vi "RX Disabled channel logic 2ch 4SPC.vi"(7 "reset":bool, 9 "input valid":bool, 10 "U32 data in":u32[](array[numeric])=[0, 0, 0, 0, 0, 0, 0, 0], 11 "enabled channels":u32) -> (1 "data ready":bool, 2 "U32 data out":u32[](array[numeric]))   [LabVIEW 2025, in "niUSRP Stream Control (DMA) v1 FPGA.lvclass"]
uses:
  niUSRP Stream Control (DMA) v1 FPGA.lvclass
  niUSRP Stream Control (DMA) v1 FPGA.lvclass/niUSRP Stream Control (DMA) v1 FPGA.ctl
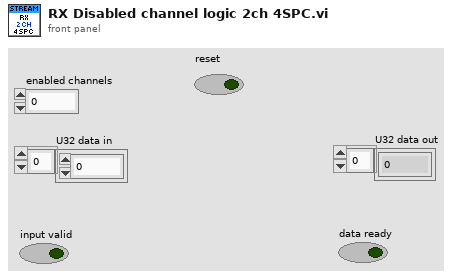
[diagram p1: front panel]
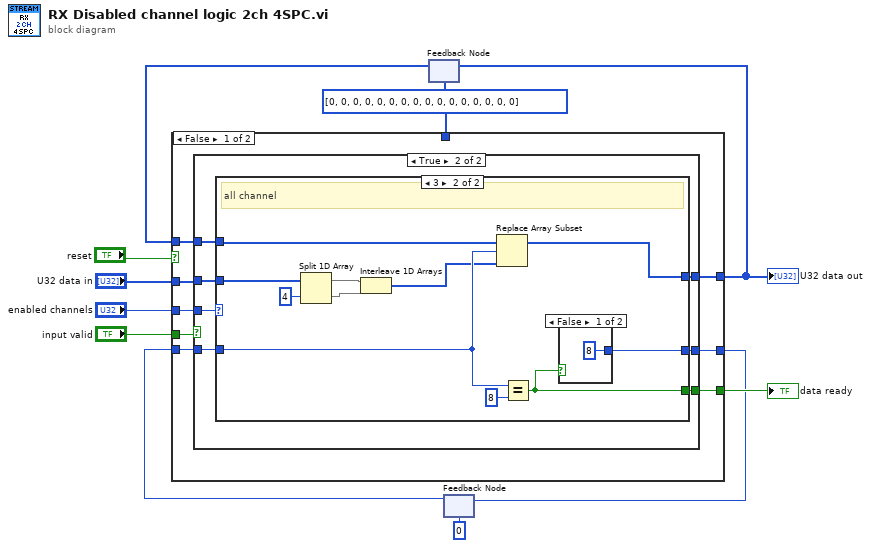
[diagram p0: block diagram]
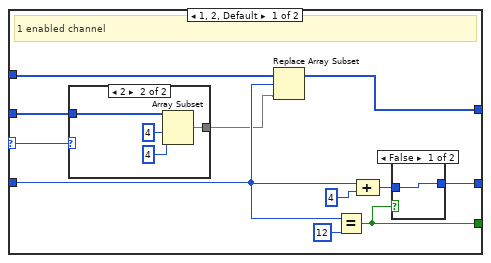
[diagram p3: hidden frame]
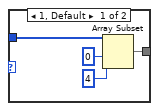
[diagram p4: hidden frame]
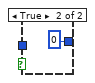
[diagram p5: hidden frame]
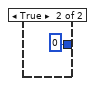
[diagram p6: hidden frame]
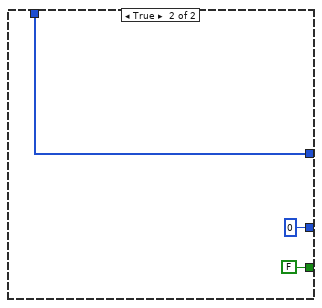
[diagram p7: hidden frame]
diagram:
  w1 = u32[] [0, 0, 0, 0, 0, 0, 0, 0, 0, 0, 0, 0, 0, 0, 0, 0]
  n1 = feedback #1(w1) -> (w11:u32[])
  n2 = feedback #2(u8 0) -> (w5:u8)
  n3 = case shown="False" "reset" {
    tunnel: w11 -> [w19 _]
    tunnel: "input valid" -> [w18 _]
    tunnel: "U32 data in" -> [w17 _]
    tunnel: [w16 w64] -> w8
    tunnel: "enabled channels" -> [w15 _]
    tunnel: w5 -> [w14 _]
    tunnel: [w13 FALSE] -> w4
    tunnel: [w12 u8 0] -> w3
    tunnel: w1 -> [_ w64]
    frame False {
      n4 = case shown="True" w18 {
        selector: w18 -> [w22 _]
        tunnel: w19 -> [w20 w29]
        tunnel: w15 -> [_ w28]
        tunnel: w17 -> [_ w27]
        tunnel: w14 -> [w21 w26]
        tunnel: [w20 w25] -> w16
        tunnel: [w21 w24] -> w12
        tunnel: [w22 w23] -> w13
        frame False {
        }
        frame True {
          n5 = case shown="3" w28 {
            selector: w28 -> [w31 _]
            tunnel: w27 -> [w32 w52]
            tunnel: [w39 w56] -> w25
            tunnel: [w35 w58] -> w23
            tunnel: w26 -> [w37 w59]
            tunnel: [w34 w57] -> w24
            tunnel: w29 -> [w38 w60]
            frame 1, 2, Default {
              # "1 enabled channel"
              n6 = case shown="2" w31 {
                tunnel: w32 -> [w42 w46]
                tunnel: [w41 w45] -> w30
                frame 1, Default {
                  n7 = Array Subset(array=w42, index=0, length=4) -> (w41:u32[])
                }
                frame 2 {
                  n8 = Array Subset(array=w46, index=4, length=4) -> (w45:u32[])
                }
              }
              n9 = Replace Array Subset(array=w38, new element=w30, index=w37) -> (w39:u32[])
              n10 = Equal?(x=w37, y=u8 12) -> (x = y?=w35:bool)
              n11 = Compound Arithmetic op=ADD(w37, u8 4 ("length")) -> (w36:u8)
              n12 = case shown="False" w35 {
                tunnel: [w49 u8 0] -> w34
                tunnel: w36 -> [w49 _]
                frame False {
                }
                frame True {
                }
              }
            }
            frame 3 {
              # "all channel"
              n13 = Split 1D Array(array=w52, index=4) -> (first subarray=w54:u32[], second subarray=w53:u32[])
              n14 = Interleave 1D Arrays(w54, w53) -> (w51:u32[])
              n15 = Replace Array Subset(array=w60, new element=w51, index=w59) -> (w56:u32[])
              n16 = Equal?(x=w59, y=u8 8) -> (x = y?=w58:bool)
              n17 = case shown="False" w58 {
                tunnel: [u8 8 u8 0] -> w57
                frame False {
                }
                frame True {
                }
              }
            }
          }
        }
      }
    }
    frame True {
    }
  }
  "data ready" <- w4
  "U32 data out" <- w8
  n18 = feedback-in #1(w8) -> ()
  n19 = feedback-in #2(w3) -> ()
